vi "writeBoolean.vi"(8 "error in (no error)":errorcluster, 10 "Data":bool, 11 "SoftwareControlledTrigger in":refnum<class "SoftwareControlledTrigger.lvclass">) -> (0 "error out":errorcluster, 3 "SoftwareControlledTrigger out":refnum<class "SoftwareControlledTrigger.lvclass">)   [LabVIEW 2016, in "SoftwareControlledTrigger.lvclass"]
uses:
  SoftwareControlledTrigger.lvclass
  SoftwareControlledTrigger.lvclass/SoftwareControlledTrigger.ctl
  <vilib>/Utility/error.llb/Error Cluster From Error Code.vi
  <vilib>/rvi/errors/niLvFpgaAdjustHostInterfaceError.vi
  <vilib>/rvi/interface/nirviReadWriteControl/nirviReadWriteControl.xnode
  NiFpgaLv.dll
  <vilib>/rvi/interface/Simulation/niFpgaSimulationCallBeginRW.vi
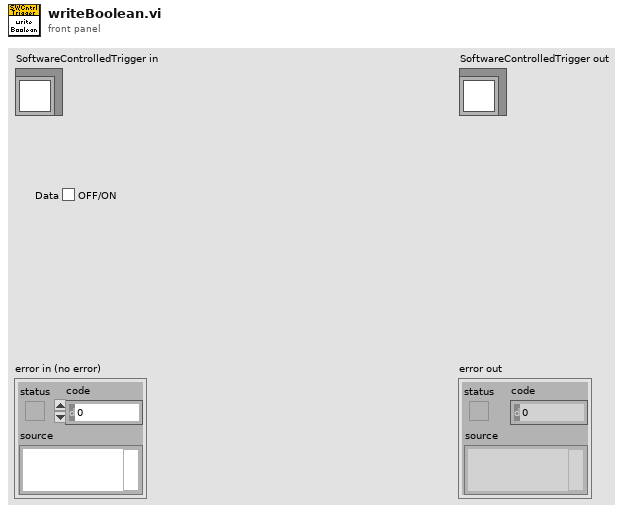
[diagram p1: front panel]
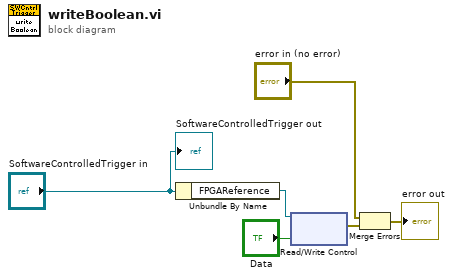
[diagram p0: block diagram]
diagram:
  n1 = Unbundle By Name("SoftwareControlledTrigger in") -> ("FPGAReference"=w6:refnum<k20>)
  n2 = xnode "Read/Write Control"("FPGA VI Reference In"=w6, "Trigger"="Data") -> ("error out"=w4:errorcluster)  [unwired: 1 in, 1 out]
  n3 = Merge Errors("error in (no error)", w4) -> (→"error out":errorcluster)
  "SoftwareControlledTrigger out" <- "SoftwareControlledTrigger in"
